vi "SetRaw.vi"(0 "reference in":refnum<class "AI.lvclass">, 5 "raw mean":dbl format="%0.2f", 11 "error in (no error)":errorcluster) -> (4 "reference out":refnum<class "AI.lvclass">, 15 "error out":errorcluster)   [LabVIEW 2019, in "AI.lvclass"]
uses:
  AI.lvclass
  C:/Users/ANENKOV_V1/Desktop/src/Proccess_class/Proccess.lvclass
  AI.lvclass/AI.ctl
  PiecedLinearScale_class/Scale_PiecedLinear.lvclass/Scale_PiecedLinear.ctl
  Proccess_class/Proccess.lvclass/Proccess.ctl
  Logger_class/Logger.lvclass/Logger.ctl
  AnalogComparator_class/AnalogComparator.lvclass/AnalogComparator.ctl
  AnalogComparator_class/SetValue.vi
  Logger_class/Enqueue Signal.vi
  Proccess_class/GetNames.vi
  Proccess_class/GetLogger.vi
  <vilib>/gmath/interp.llb/Interpolate 1D.vi
  <vilib>/Utility/error.llb/Error Cluster From Error Code.vi
  AnalogComparator_class/SendToDb.vi
  PiecedLinearScale_class/Scale_PiecedLinear.lvclass
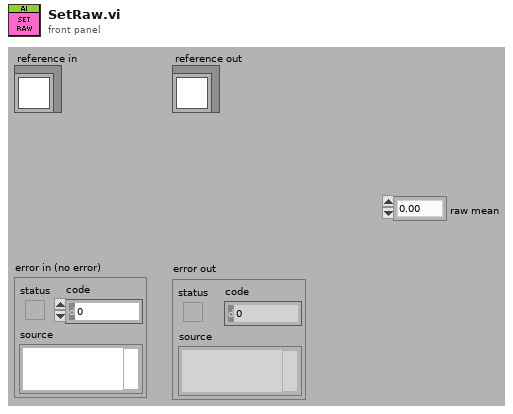
[diagram p1: front panel]
types:
  T1 = typedef "Data Avr.ctl" = cluster{"data":dbl[], "indx":i32}
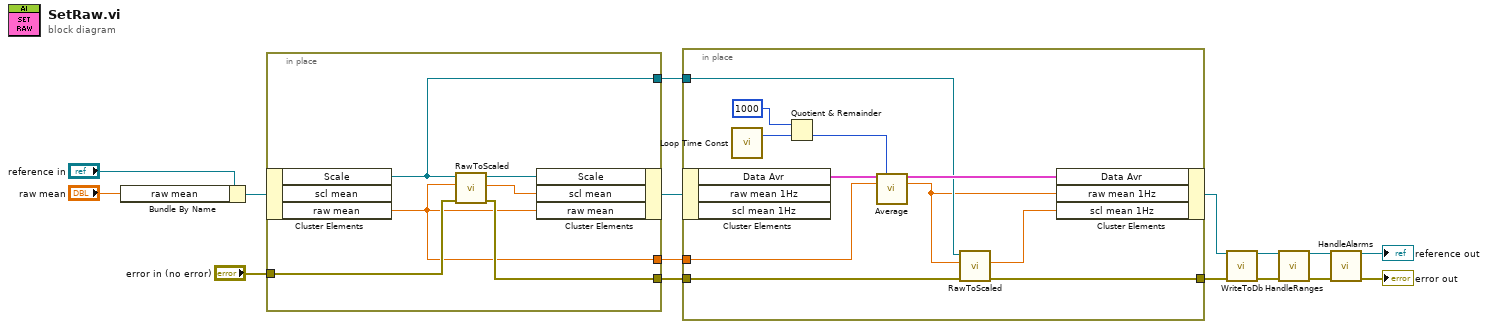
[diagram p0: block diagram]
diagram:
  n1 = Bundle By Name(cluster="reference in", "raw mean"="raw mean") -> (w6:refnum<class "AI.lvclass">)
  n2 = in-place {
    in-place-border: [w17] -> w12
    in-place-border: "error in (no error)" -> [w22]
    in-place-border: [w21] -> w10
    in-place-border: [w18] -> w9
    n3 = in-place-cluster #1(w6) -> ("Scale"=w18:refnum<class "Scale_PiecedLinear.lvclass">, "raw mean"=w17:dbl)  [unwired: 1 out]
    n4 = call "RawToScaled.vi"("error in (no error)"=w22, "RAW"=w17, "PiecedLinearScale in"=w18) -> ("error out"=w21:errorcluster, "Scaled"=w19:dbl, "PiecedLinearScale out"=w20:refnum<class "Scale_PiecedLinear.lvclass">)  [unwired: 6 in]
    n5 = in-place-cluster #1("Scale"=w20, "scl mean"=w19, "raw mean"=w17) -> (w13:refnum<class "AI.lvclass">)
  }
  n6 = in-place {
    in-place-border: w12 -> [w31]
    in-place-border: w10 -> [w27]
    in-place-border: [w26] -> w2
    in-place-border: w9 -> [w30]
    n7 = in-place-cluster #2(w13) -> ("Data Avr"=w33:T1)  [unwired: 2 out]
    n8 = call "Loop Time Const.vi"() -> ("loop time ms"=w25:i64)  [unwired: 3 in]
    n9 = Quotient & Remainder(x=i64 1000, y=w25) -> (floor(x/y)=w23:i64)  [unwired: 1 out]
    n10 = call "Average.vi"("Data Avr in"=w33, "Size"=w23, "VALUE"=w31) -> ("Data Avr out"=w32:T1, "AVR"=w29:dbl)  [unwired: 11 in]
    n11 = call "RawToScaled.vi"("error in (no error)"=w27, "RAW"=w29, "PiecedLinearScale in"=w30) -> ("error out"=w26:errorcluster, "Scaled"=w28:dbl)  [unwired: 6 in, 1 out]
    n12 = in-place-cluster #2("Data Avr"=w32, "raw mean 1Hz"=w29, "scl mean 1Hz"=w28) -> (w1:refnum<class "AI.lvclass">)
  }
  n13 = call "WriteToDb.vi"("reference in"=w1, "error in (no error)"=w2) -> ("reference out"=w3:refnum<class "AI.lvclass">, "error out"=w4:errorcluster)  [unwired: 12 in]
  n14 = call "HandleRanges.vi"("reference in"=w3, "error in (no error)"=w4) -> ("reference out"=w8:refnum<class "AI.lvclass">, "error out"=w7:errorcluster)  [unwired: 12 in]
  n15 = call "HandleAlarms.vi"("reference in"=w8, "error in (no error)"=w7) -> ("reference out"=→"reference out":refnum<class "AI.lvclass">, "error out"=→"error out":errorcluster)  [unwired: 12 in]
